vi "Go to MHL Case MHLC.vi"(8 "error in (no error)":errorcluster, 10 "Data in":variant, 11 "AppMgr in":refnum<class "Application Manager.lvclass">) -> (0 "error out":errorcluster, 3 "AppMgr out":refnum<class "Application Manager.lvclass">)   [LabVIEW 2017, in "Application Manager.lvclass"]
doc: "Show the selected MHL on the block diagram of the Main VI of the selected Worker"
uses:
  Application Manager.lvclass
  rqp_Go to MHL Case.ctl
  Common VIs/DC_UID.ctl
  Application Manager.lvclass/Application Manager.ctl
  rsp_Go to MHL Case - Response.ctl
  <vilib>/Utility/error.llb/Error Cluster From Error Code.vi
  <vilib>/ErrorRing/Error Ring.xnode
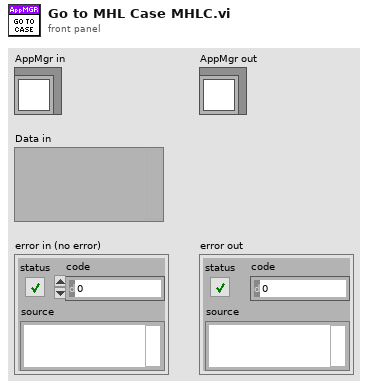
[diagram p1: front panel]
types:
  T1 = typedef "Application Manager.lvclass/rqp_Go to MHL Case.ctl" = cluster{"DC_UID":T2, "Worker ID":string, "Case Name":string}
  T2 = typedef "DC_UID.ctl" = string
  T3 = typedef "Application Manager.lvclass/Debug Client Data.ctl" = cluster{"DC_UID":T2, "IP Address":string, "Worker Data":T4[], "Connected":bool}
  T4 = typedef "Application Manager.lvclass/Worker Data.ctl" = cluster{"ID":string, "VI Ref":refnum<vi>, "VI Path":path, "CloneID":string, "Type":T5, "Worker Status":string}
  T5 = typedef "Workers.lvlib/Worker.lvclass/Worker Type.ctl" = enum16{"SL", "DL"}
  T6 = typedef "Application Manager.lvclass/rsp_Go to MHL Case - Response.ctl" = cluster{"DC_UID":T2, "VI Path":path, "Case Name":string}
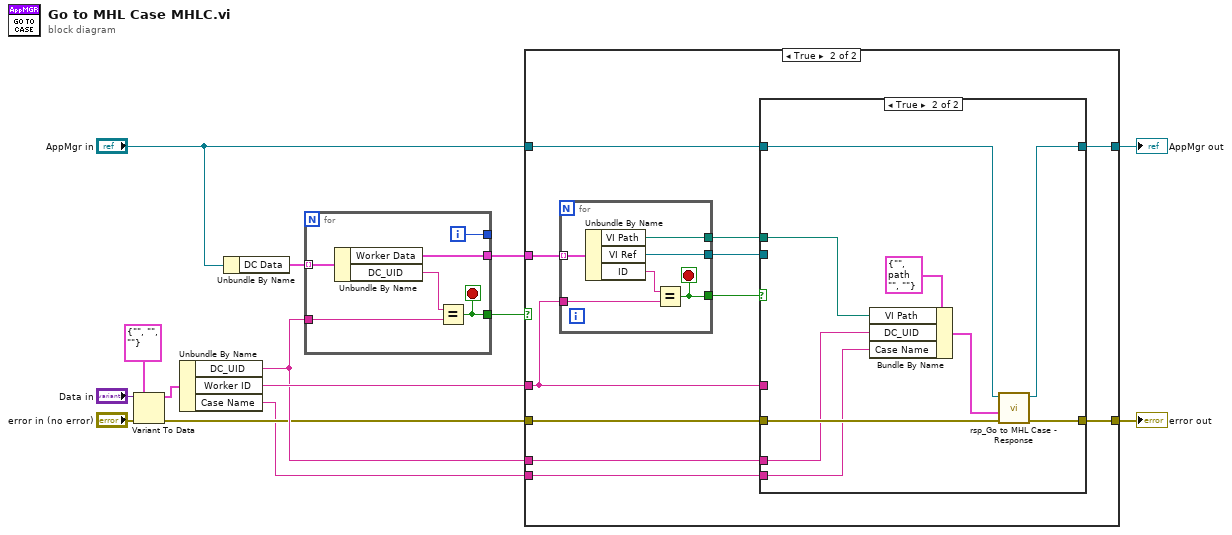
[diagram p0: block diagram]
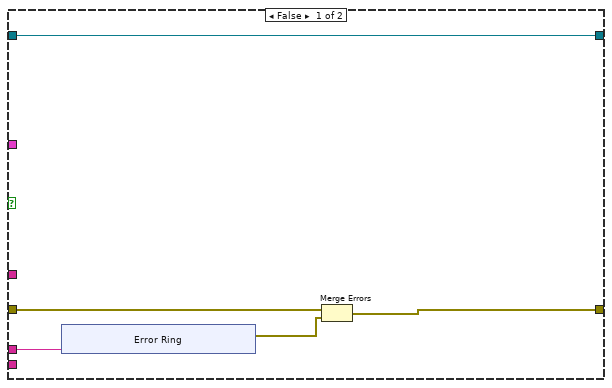
[diagram p2: hidden frame]
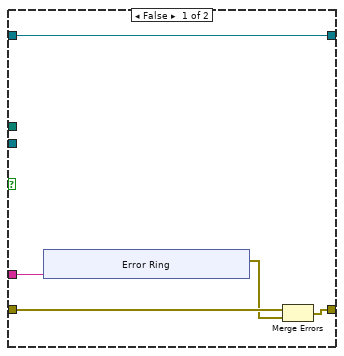
[diagram p3: hidden frame]
diagram:
  n1 = Variant To Data(error in="error in (no error)", type=T1 {"DC_UID"="", "Worker ID"="", "Case Name"=""} ("Data"), Variant="Data in") -> (data=w5:T1, error out=w9:errorcluster)
  n2 = Unbundle By Name(w5) -> ("DC_UID"=w12:T2, "Worker ID"=w14:string, "Case Name"=w1:string)
  n3 = Unbundle By Name("AppMgr in") -> ("DC Data"=w6:T3[])
  n4 = for {
    tunnel: w6 -> [w17] mode=indexing
    tunnel: [w19] -> w11
    tunnel: [w18] -> _
    tunnel: [w15] -> w13
    tunnel: w12 -> [w16]
    i -> [w18]
    stop <- w19 stop-if-true
    n5 = Unbundle By Name(w17) -> ("Worker Data"=w15:T4[], "DC_UID"=w20:T2)
    n6 = Equal?(x=w20, y=w16) -> (x = y?=w19:bool)
  }
  n7 = case shown="True" w11 {
    tunnel: "AppMgr in" -> [w25 w40]
    tunnel: [w25 w39] -> w8
    tunnel: w9 -> [w24 w43]
    tunnel: [w23 w41] -> w10
    tunnel: w12 -> [w21 w38]
    tunnel: w13 -> [_ w42]
    tunnel: w14 -> [_ w34]
    tunnel: w1 -> [_ w33]
    frame False {
      n8 = xnode "Error Ring"("parameter 0"=w21) -> ("error out"=w22:errorcluster)
      n9 = Merge Errors(w24, w22) -> (w23:errorcluster)
    }
    frame True {
      n10 = for {
        tunnel: w42 -> [w70] mode=indexing
        tunnel: w34 -> [w68]
        tunnel: [w67] -> w35
        tunnel: [w66] -> w36
        tunnel: [w65] -> w37
        stop <- w67 stop-if-true
        n11 = Unbundle By Name(w70) -> ("VI Path"=w66:path, "VI Ref"=w65:refnum<vi>, "ID"=w69:string)
        n12 = Equal?(x=w69, y=w68) -> (x = y?=w67:bool)
      }
      n13 = case shown="True" w35 {
        tunnel: w43 -> [w48 w64]
        tunnel: [w47 w63] -> w41
        tunnel: w40 -> [w46 w62]
        tunnel: [w46 w61] -> w39
        tunnel: w38 -> [_ w59]
        tunnel: w37 -> [_ _]
        tunnel: w36 -> [_ w58]
        tunnel: w34 -> [w44 _]
        tunnel: w33 -> [_ w56]
        frame False {
          n14 = xnode "Error Ring"("parameter 0"=w44) -> ("error out"=w45:errorcluster)
          n15 = Merge Errors(w48, w45) -> (w47:errorcluster)
        }
        frame True {
          n16 = Bundle By Name(cluster=T6 {"DC_UID"="", "VI Path"=path "", "Case Name"=""} ("Data in"), "VI Path"=w58, "DC_UID"=w59, "Case Name"=w56) -> (w57:T6)
          n17 = call "rsp_Go to MHL Case - Response.vi"("error in"=w64, "Data in"=w57, "Application Manager in"=w62) -> ("error out"=w63:errorcluster, "dup Application Manager out"=w61:refnum<class "Application Manager.lvclass">)  [unwired: 7 in]
        }
      }
    }
  }
  "error out" <- w10
  "AppMgr out" <- w8
